vi "SA_GetStatus_S.vi"(5 "channelIndex":u32, 7 "systemIndex":u32, 8 "error in (no error)":errorcluster) -> (0 "error out":errorcluster, 3 "status":T1(ring))   [LabVIEW 2013]
doc: "<B>Description:</B>\nReturns the current movement status of a positioner (see the appendix for a list of movement status codes). This function can be used to check whether a previously issued movement command has been completed.\n<B>Parameters:</B>\n<B>- systemIndex</B> (unsigned 32bit), input - Selects the system. The index is zero based.\n<B>- channelIndex</B> (unsigned 32bit), input - Selects the channel of the selected system. The index is zero based.\n<B>- status</B> (unsigned 32bit), output - If the call was successful this value holds the current status of the positioner. Please refer to the 'Programmer's Guide' for a list of status codes."
uses:
  MCSControl.dll
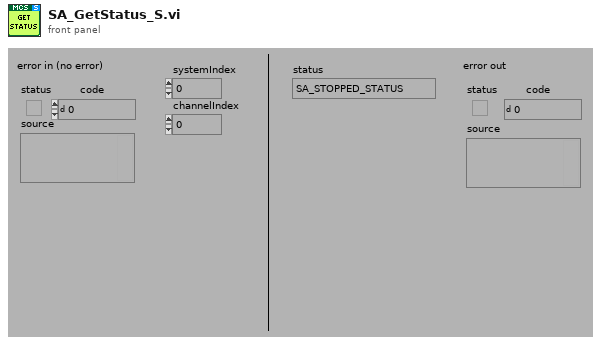
[diagram p1: front panel]
types:
  T1 = enum32{"SA_STOPPED_STATUS", "SA_STEPPING_STATUS", "SA_SCANNING_STATUS", "SA_HOLDING_STATUS", "SA_TARGET_STATUS", "SA_MOVE_DELAY_STATUS", "SA_CALIBRATING_STATUS", "SA_FINDING_REF_STATUS", "SA_OPENING_STATUS"}
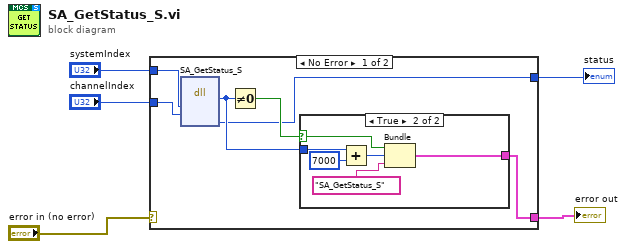
[diagram p0: block diagram]
diagram:
  n1 = case shown="No Error" "error in (no error)" {
    selector: "error in (no error)" -> [_ w18]
    tunnel: [w9 w18] -> w4
    tunnel: "systemIndex" -> [w8 _]
    tunnel: "channelIndex" -> [w7 _]
    tunnel: [w6 _] -> w1
    frame No Error {
      n2 = dll-call lib="MCSControl.dll" fn="SA_GetStatus_S"("systemIndex"=w8, "channelIndex"=w7) -> ("return type"=w10:u32, "status"=w6:u32)  [unwired: 6 in, 2 out]
      n3 = Not Equal To 0?(x=w10) -> (x != 0?=w11:bool)
      n4 = case shown="True" w11 {
        selector: w11 -> [_ w14]
        tunnel: w10 -> [_ w17]
        tunnel: [_ w12] -> w9
        frame False {
        }
        frame True {
          n5 = Add(x=w17, y=u32 7000) -> (x+y=w15:u32)
          n6 = Bundle(w14, w15, "source"="SA_GetStatus_S") -> (w12:cluster{bool, u32, "source":string})  [unwired: 1 in]
        }
      }
    }
    frame Error {
    }
  }
  "error out" <- w4
  "status" <- w1
